vi "startAcq.vi"(8 "error in (no error)":errorcluster, 10 "Array 3":refnum<class "RADEBase.lvclass">[](array[class]), 11 "DataParameters":T2(array[cluster])) -> (2 "Array 2":refnum<class "RADEBase.lvclass">[](array[class]), 3 "Array":errorcluster[](array[cluster]))   [LabVIEW 2014]
uses:
  <userlib>/_RADE/RIO/RADEBase/classes/RADEBase/RADEBase.lvclass
panel:
  out "Array 4":T1(array[cluster])
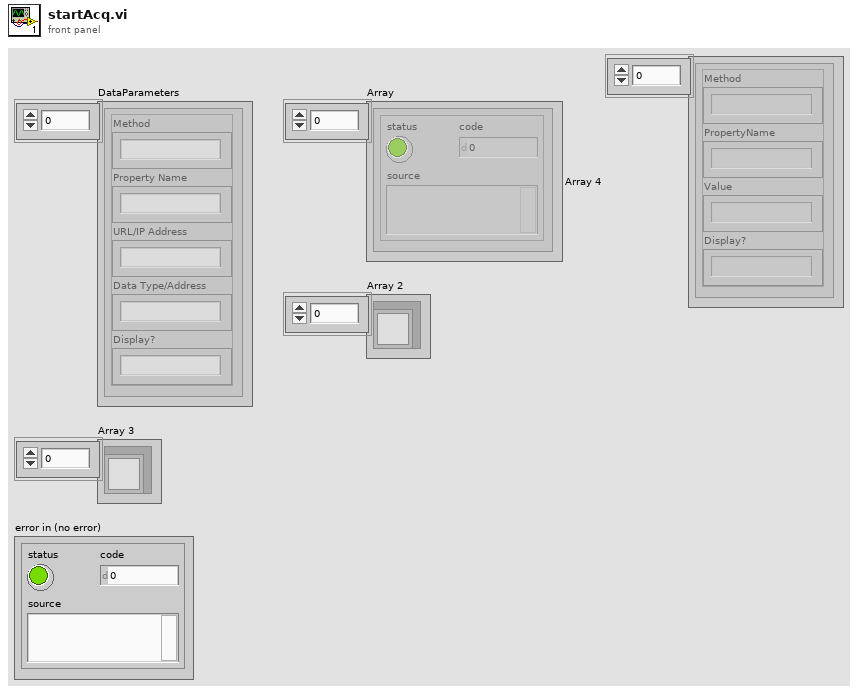
[diagram p1: front panel]
types:
  T1 = cluster{"Method":string, "PropertyName":string, "Value":string, "Display?":string}[]
  T2 = cluster{"Method":string, "Property Name":string, "URL/IP Address":string, "Data Type/Address":string, "Display?":string}[]
  T3 = cluster{"Method":string, "PropertyName":string, "Value":string, "Display?":string}
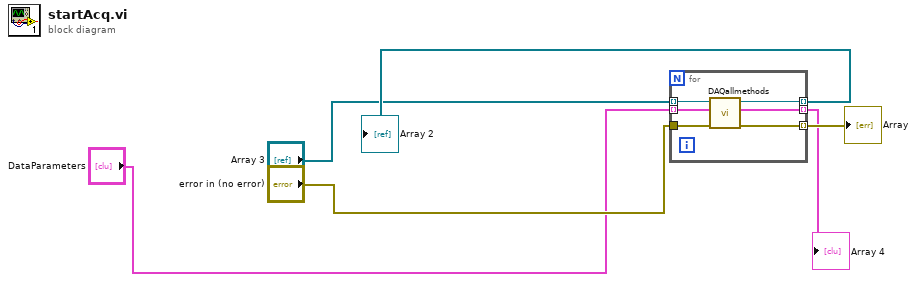
[diagram p0: block diagram]
diagram:
  n1 = for {
    tunnel: "Array 3" -> [w12] mode=indexing
    tunnel: "DataParameters" -> [w11] mode=indexing
    tunnel: [w10] -> w4 mode=indexing
    tunnel: "error in (no error)" -> [w9]
    tunnel: [w8] -> w5 mode=indexing
    tunnel: [w7] -> w1 mode=indexing
    n2 = call "DAQallmethods.vi"("error in"=w9, "InputParameters"=w11, "fromINIT"=w12) -> ("error out"=w8:errorcluster, "DataPack"=w7:T3, "toExit"=w10:refnum<class "RADEBase.lvclass">)  [unwired: 6 in]
  }
  "Array" <- w5
  "Array 2" <- w4
  "Array 4" <- w1
